vi "Get Cursor.vi"(8 "error in (no error)":errorcluster, 11 "SQLite3LV Connection in":refnum<class "sqlite3.lvclass">) -> (0 "error out":errorcluster, 2 "SQLite3LV Cursor":refnum<class "cursor.lvclass">, 3 "SQLite3LV Connection out":refnum<class "sqlite3.lvclass">)   [LabVIEW 2014, in "SQLite3LV.lvlib" / "sqlite3.lvclass"]
doc: "Creates a SQLite3LV Cursor from an active database connection.\n\nMultiple cursors can be created for a single connection.\n\nOnly one cursor should be used to access the database connection at any time.\n\nClient code is required to implement all synchronization to ensure that the database connection is used by only one thread at a time. \n\nThe helper methods \"Get Lock\" will return a memory reference lock for the database connection. This lock may be use to synchronize access to the database connection from multiple threads or subVIs."
uses:
  sqlite3.lvclass
  Cursor Class/cursor.lvclass
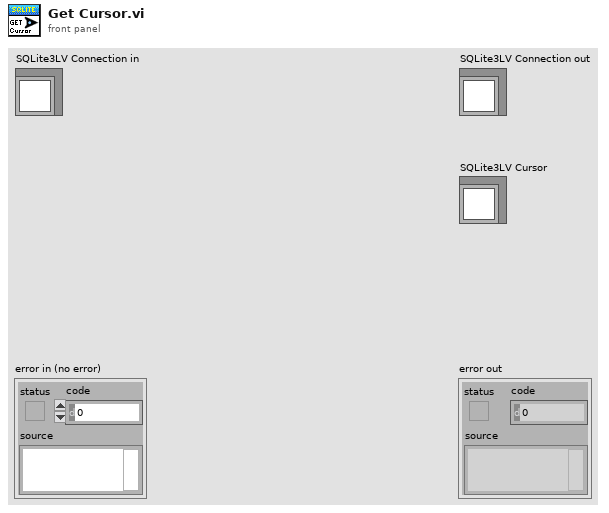
[diagram p1: front panel]
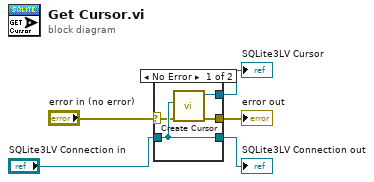
[diagram p0: block diagram]
diagram:
  n1 = case shown="No Error" "error in (no error)" {
    selector: "error in (no error)" -> [w8 w11]
    tunnel: [w7 w11] -> w4
    tunnel: [w9 w10] -> w2
    tunnel: "SQLite3LV Connection in" -> [w9 w10]
    tunnel: [w6 _] -> w1
    frame No Error {
      n2 = call "Create Cursor.vi"("error in (no error)"=w8, "SQLite3LV Connection"=w9) -> ("error out"=w7:errorcluster, "SQLite3LV Cursor out"=w6:refnum<class "cursor.lvclass">)  [unwired: 8 in]
    }
    frame Error {
    }
  }
  "error out" <- w4
  "SQLite3LV Connection out" <- w2
  "SQLite3LV Cursor" <- w1
